vi "butterfly_valve_subVI_V2.vi"(6 "% open / desired pressure / pressure mode":T1, 8 "error in (no error)":errorcluster, 11 "VISA Refnum in":refnum<visa-resource-name>) -> (0 "error out":errorcluster, 3 "VISA Refnum out":refnum<visa-resource-name>, 5 "Valve position (%)":dbl)   [LabVIEW 2014]
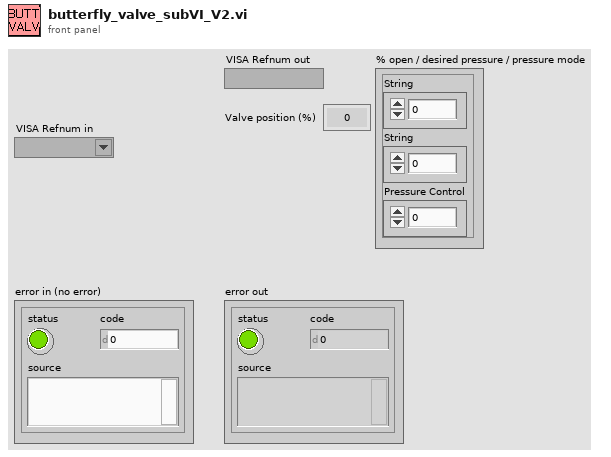
[diagram p1: front panel]
types:
  T1 = cluster{"String":dbl, "String":dbl, "Pressure Control":u32}
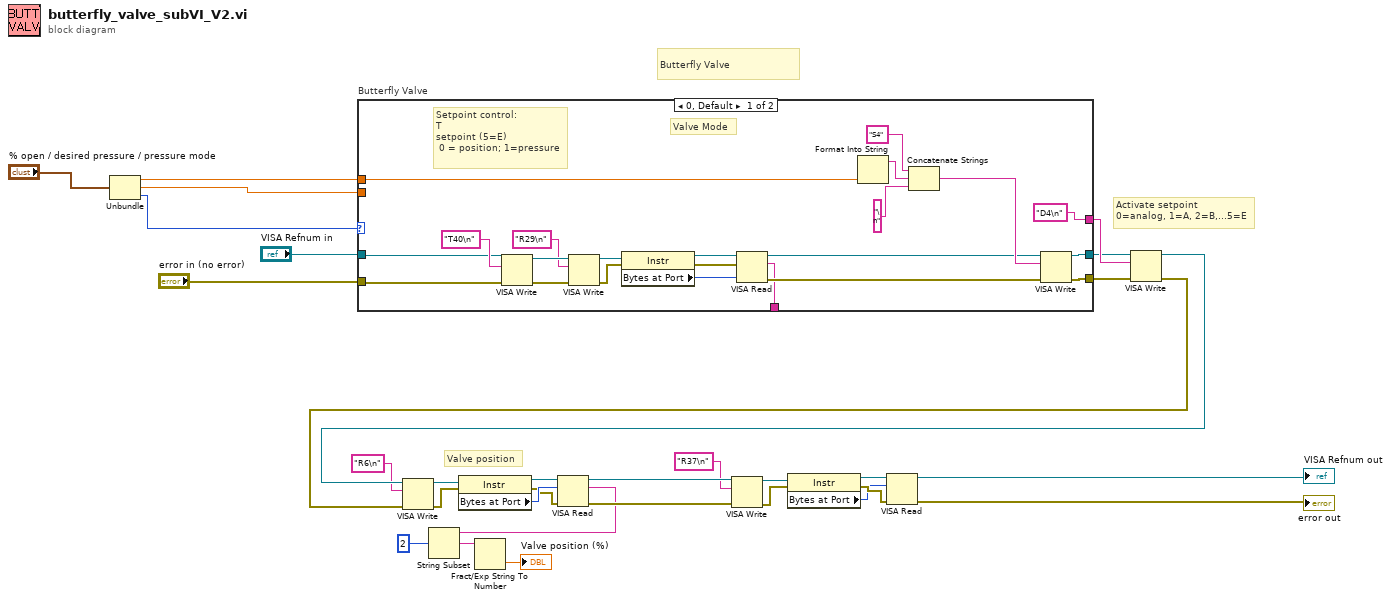
[diagram p0: block diagram]
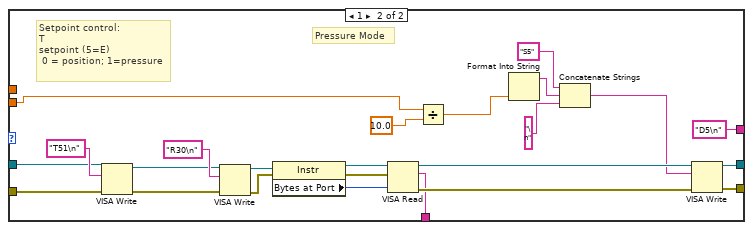
[diagram p2: hidden frame]
diagram:
  # "Activate setpoint \n0=analog, 1=A, 2=B,...5=E"
  # "Valve position"
  # "Butterfly Valve"
  n1 = Unbundle("% open / desired pressure / pressure mode") -> ("String"=w1:dbl, "String"=w2:dbl, "Pressure Control"=w3:u32)
  n2 = case "Butterfly Valve" shown="0, Default" w3 {
    tunnel: "VISA Refnum in" -> [w38 w59]
    tunnel: "error in (no error)" -> [w37 w60]
    tunnel: [w36 w62] -> w23
    tunnel: [w35 w61] -> w24
    tunnel: [w34 w58] -> _
    tunnel: ["D4\n" ("write buffer") "D5\n" ("write buffer")] -> w25
    tunnel: w2 -> [_ w54]
    tunnel: w1 -> [w32 _]
    frame 0, Default {
      # "Valve Mode"
      # "Setpoint control:\nT\nsetpoint (5=E)\n 0 = position; 1=pressure"
      n3 = VISA Write(VISA resource name=w38, write buffer="T40\n", error in (no error)=w37) -> (VISA resource name out=w49:refnum<visa-resource-name>, error out=w47:errorcluster)  [unwired: 1 out]
      n4 = VISA Write(VISA resource name=w49, write buffer="R29\n", error in (no error)=w47) -> (VISA resource name out=w42:refnum<visa-resource-name>, error out=w43:errorcluster)  [unwired: 1 out]
      n5 = property class="Instr"(reference=w42, error in=w43) -> (reference out=w40:refnum<visa-resource-name>, error out=w41:errorcluster, "Bytes at Port"=w48:u32)
      n6 = VISA Read(VISA resource name=w40, byte count=w48, error in (no error)=w41) -> (VISA resource name out=w46:refnum<visa-resource-name>, read buffer=w34:string, error out=w45:errorcluster)  [unwired: 1 out]
      n7 = Format Into String(w32) -> (resulting string=w53:string)  [unwired: 3 in, 1 out]
      n8 = Concatenate Strings("S4" ("string"), w53, "\n" ("string")) -> (w51:string)
      n9 = VISA Write(VISA resource name=w46, write buffer=w51, error in (no error)=w45) -> (VISA resource name out=w36:refnum<visa-resource-name>, error out=w35:errorcluster)  [unwired: 1 out]
    }
    frame 1 {
      # "Pressure Mode"
      # "Setpoint control:\nT\nsetpoint (5=E)\n 0 = position; 1=pressure"
      n10 = VISA Write(VISA resource name=w59, write buffer="T51\n", error in (no error)=w60) -> (VISA resource name out=w67:refnum<visa-resource-name>, error out=w69:errorcluster)  [unwired: 1 out]
      n11 = VISA Write(VISA resource name=w67, write buffer="R30\n", error in (no error)=w69) -> (VISA resource name out=w74:refnum<visa-resource-name>, error out=w73:errorcluster)  [unwired: 1 out]
      n12 = property class="Instr"(reference=w74, error in=w73) -> (reference out=w76:refnum<visa-resource-name>, error out=w75:errorcluster, "Bytes at Port"=w68:u32)
      n13 = VISA Read(VISA resource name=w76, byte count=w68, error in (no error)=w75) -> (VISA resource name out=w70:refnum<visa-resource-name>, read buffer=w58:string, error out=w71:errorcluster)  [unwired: 1 out]
      n14 = Divide(x=w54, y=10.0) -> (x/y=w55:dbl)
      n15 = Format Into String(w55) -> (resulting string=w63:string)  [unwired: 3 in, 1 out]
      n16 = Concatenate Strings("S5" ("string"), w63, "\n" ("string")) -> (w65:string)
      n17 = VISA Write(VISA resource name=w70, write buffer=w65, error in (no error)=w71) -> (VISA resource name out=w62:refnum<visa-resource-name>, error out=w61:errorcluster)  [unwired: 1 out]
    }
  }
  n18 = VISA Write(VISA resource name=w23, write buffer=w25, error in (no error)=w24) -> (VISA resource name out=w27:refnum<visa-resource-name>, error out=w28:errorcluster)  [unwired: 1 out]
  n19 = VISA Write(VISA resource name=w27, write buffer="R6\n", error in (no error)=w28) -> (VISA resource name out=w9:refnum<visa-resource-name>, error out=w10:errorcluster)  [unwired: 1 out]
  n20 = property class="Instr"(reference=w9, error in=w10) -> (reference out=w6:refnum<visa-resource-name>, error out=w7:errorcluster, "Bytes at Port"=w8:u32)
  n21 = VISA Read(VISA resource name=w6, byte count=w8, error in (no error)=w7) -> (VISA resource name out=w20:refnum<visa-resource-name>, read buffer=w11:string, error out=w21:errorcluster)  [unwired: 1 out]
  n22 = String Subset(string=w11, offset (0)=2) -> (substring=w13:string)  [unwired: 1 in]
  n23 = Fract/Exp String To Number(string=w13) -> (number=→"Valve position (%)":dbl)  [unwired: 3 in, 1 out]
  n24 = VISA Write(VISA resource name=w20, write buffer="R37\n", error in (no error)=w21) -> (VISA resource name out=w15:refnum<visa-resource-name>, error out=w14:errorcluster)  [unwired: 1 out]
  n25 = property class="Instr"(reference=w15, error in=w14) -> (reference out=w18:refnum<visa-resource-name>, error out=w17:errorcluster, "Bytes at Port"=w16:u32)
  n26 = VISA Read(VISA resource name=w18, byte count=w16, error in (no error)=w17) -> (VISA resource name out=→"VISA Refnum out":refnum<visa-resource-name>, error out=→"error out":errorcluster)  [unwired: 2 out]
